vi "RemoveRectFromScreen.vi"(8 "IntensityArray_IN":u8[][](array[numeric]), 11 "Position":T1) -> (0 "IntensityArray_OUT":u8[][](array[numeric]))   [LabVIEW 2022 SP3]
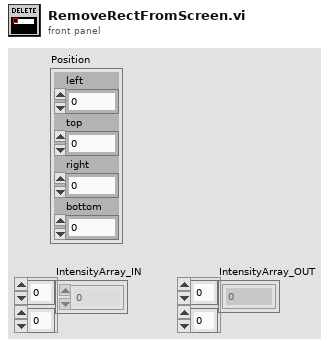
[diagram p1: front panel]
types:
  T1 = cluster{"left":i16, "top":i16, "right":i16, "bottom":i16}
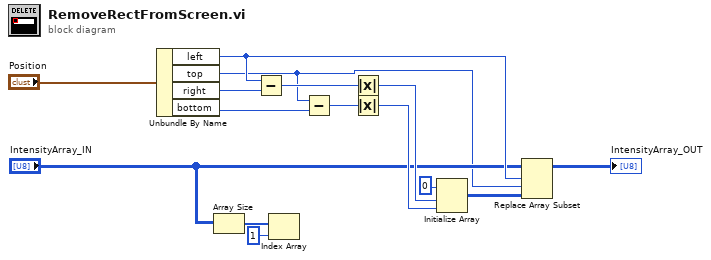
[diagram p0: block diagram]
diagram:
  n1 = Unbundle By Name("Position") -> ("left"=w11:i16, "top"=w2:i16, "right"=w10:i16, "bottom"=w6:i16)
  n2 = Array Size(array="IntensityArray_IN") -> (size(s)=w4:i32[])
  n3 = Subtract(x=w11, y=w10) -> (x-y=w13:i16)
  n4 = Index Array(array=w4, index=1) -> ()  [unwired: 1 out]
  n5 = Subtract(x=w2, y=w6) -> (x-y=w12:i16)
  n6 = Absolute Value(x=w13) -> (abs(x)=w8:i16)
  n7 = Absolute Value(x=w12) -> (abs(x)=w7:i16)
  n8 = Initialize Array(u8 0 ("element"), w8, w7) -> (w14:u8[][])
  n9 = Replace Array Subset(array="IntensityArray_IN", new element=w14, index (row)=w11, index (col)=w2) -> (→"IntensityArray_OUT":u8[][])
